vi "Set Main Pane Reference.vi"(8 "error in (no error)":errorcluster, 10 "Main Pane":refnum<vi>, 11 "Flex UI in":refnum<class "Flex UI.lvclass">) -> (0 "error out":errorcluster, 3 "Flex UI out":refnum<class "Flex UI.lvclass">)   [LabVIEW 2016, in "Flex UI.lvclass"]
uses:
  Flex UI.lvclass
  Flex UI.lvclass/Flex UI.ctl
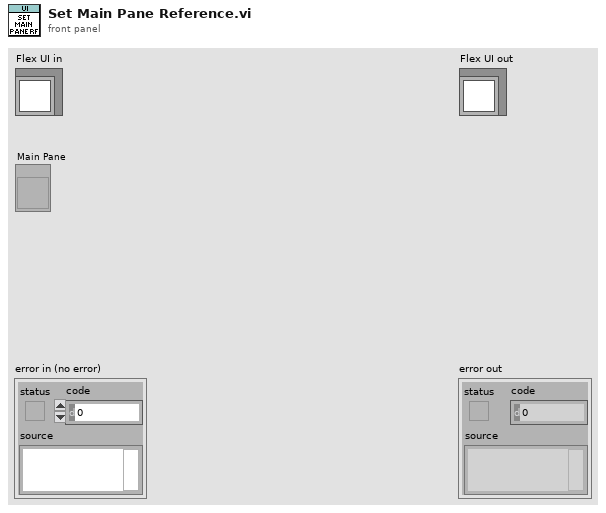
[diagram p1: front panel]
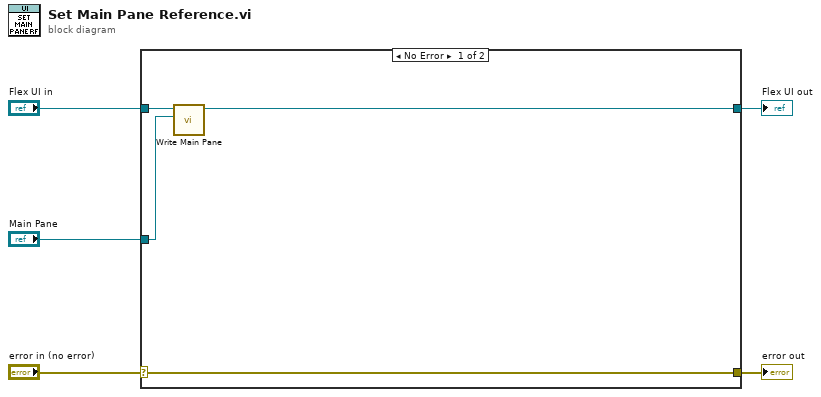
[diagram p0: block diagram]
diagram:
  n1 = case shown="No Error" "error in (no error)" {
    selector: "error in (no error)" -> [w8 w11]
    tunnel: [w8 w11] -> w4
    tunnel: [w7 w10] -> w2
    tunnel: "Flex UI in" -> [w9 w10]
    tunnel: "Main Pane" -> [w6 _]
    frame No Error {
      n2 = call "Write Main Pane.vi"("Main Pane"=w6, "Flex UI in"=w9) -> ("Flex UI out"=w7:refnum<class "Flex UI.lvclass">)  [unwired: 9 in]
    }
    frame Error {
    }
  }
  "error out" <- w4
  "Flex UI out" <- w2
